vi "PCO_RecorderSaveImage_B8.vi"(0 "pImgBuf":u8[][](array[numeric])=array1x4097[4097 elements], 1 "wWidth":u16, 2 "wHeight":u16, 3 "szFilePath":path, 5 "error in (no error)":errorcluster {"code" format="%x"}, 6 "isColor":bool, 8 "bIsBitmap":bool, 9 "PCO_METADATA_STRUCT":T1, 10 "bOverwrite":bool) -> (14 "ErrorMessage":i32 format="%x", 19 "error out":errorcluster {"code" format="%x"})   [LabVIEW 2019, in "Recorder.lvlib"]
doc: "int WINAPI PCO_RecorderSaveImage(void* pImgBuf, WORD wWidth, WORD wHeight, const char* cFileType, bool bIsBitmap, const char* szFilePath, bool bOverwrite, PCO_METADATA_STRUCT* strMetadata);"
uses:
  Recorder.lvlib
  pco.sdk/Structures/Structures.lvlib
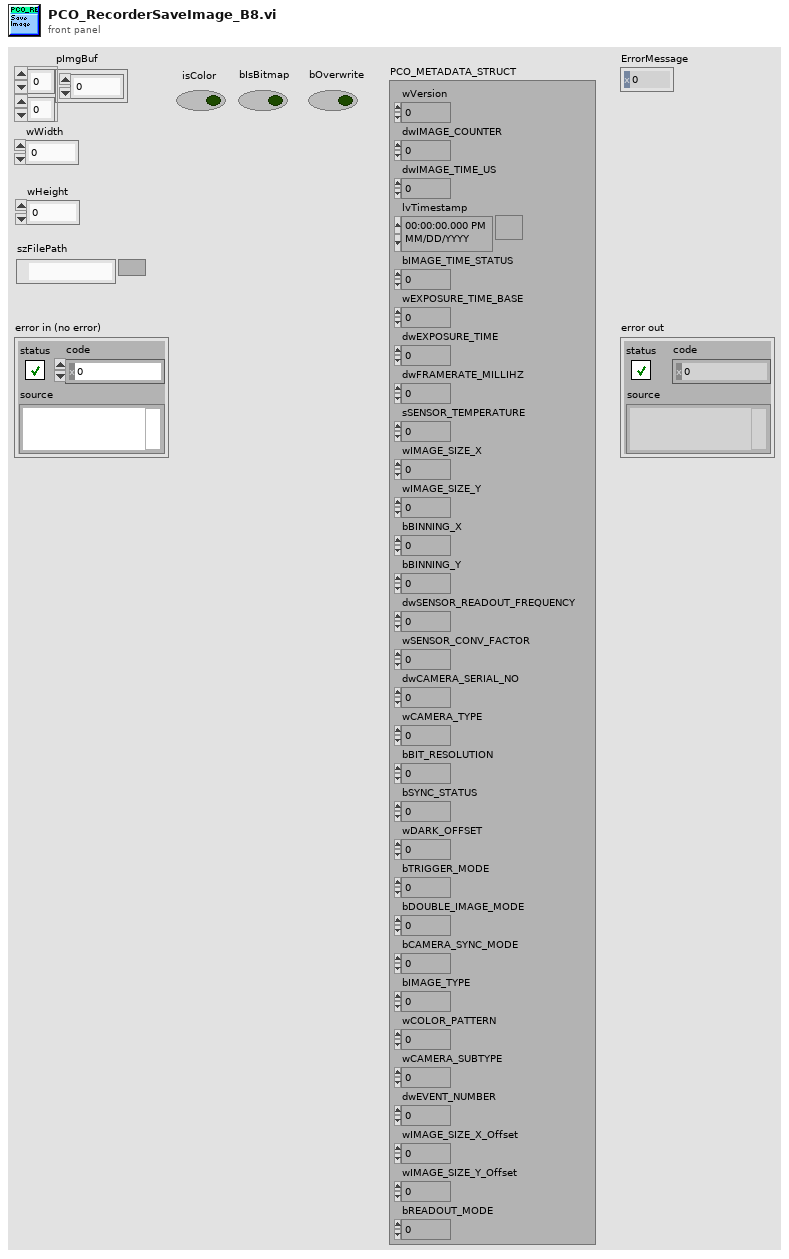
[diagram p1: front panel]
types:
  T1 = cluster{"wVersion":u16, "dwIMAGE_COUNTER":u32, "dwIMAGE_TIME_US":u32, "lvTimestamp":timestamp, "bIMAGE_TIME_STATUS":u8, "wEXPOSURE_TIME_BASE":u16, "dwEXPOSURE_TIME":u32, "dwFRAMERATE_MILLIHZ":u32, "sSENSOR_TEMPERATURE":i16, "wIMAGE_SIZE_X":u16, "wIMAGE_SIZE_Y":u16, "bBINNING_X":u8, "bBINNING_Y":u8, "dwSENSOR_READOUT_FREQUENCY":u32, "wSENSOR_CONV_FACTOR":u16, "dwCAMERA_SERIAL_NO":u32, "wCAMERA_TYPE":u16, "bBIT_RESOLUTION":u8, "bSYNC_STATUS":u8, "wDARK_OFFSET":u16, "bTRIGGER_MODE":u8, "bDOUBLE_IMAGE_MODE":u8, "bCAMERA_SYNC_MODE":u8, "bIMAGE_TYPE":u8, "wCOLOR_PATTERN":u16, "wCAMERA_SUBTYPE":u16, "dwEVENT_NUMBER":u32, "wIMAGE_SIZE_X_Offset":u16, "wIMAGE_SIZE_Y_Offset":u16, "bREADOUT_MODE":u8}
  T2 = typedef "LVDateTimeRec.ctl" = cluster{"fractional second":dbl, "second":i32, "minute":i32, "hour":i32, "day of month":i32, "month":i32, "year":i32, "day of week":i32, "day of year":i32, "DST":i32}
  T3 = cluster{"wSize":u16, "wVersion":u16, "bIMAGE_COUNTER_BCD":cluster{u8, u8, u8, u8}, "bIMAGE_TIME_US_BCD":cluster{u8, u8, u8}, "bIMAGE_TIME_SEC_BCD":u8, "bIMAGE_TIME_MIN_BCD":u8, "bIMAGE_TIME_HOUR_BCD":u8, "bIMAGE_TIME_DAY_BCD":u8, "bIMAGE_TIME_MON_BCD":u8, "bIMAGE_TIME_YEAR_BCD":u8, "bIMAGE_TIME_STATUS":u8, "wEXPOSURE_TIME_BASE":u16, "dwEXPOSURE_TIME":u32, "dwFRAMERATE_MILLIHZ":u32, "sSENSOR_TEMPERATURE":i16, "wIMAGE_SIZE_X":u16, "wIMAGE_SIZE_Y":u16, "bBINNING_X":u8, "bBINNING_Y":u8, "dwSENSOR_READOUT_FREQUENCY":u32, "wSENSOR_CONV_FACTOR":u16, "dwCAMERA_SERIAL_NO":u32, "wCAMERA_TYPE":u16, "bBIT_RESOLUTION":u8, "bSYNC_STATUS":u8, "wDARK_OFFSET":u16, "bTRIGGER_MODE":u8, "bDOUBLE_IMAGE_MODE":u8, "bCAMERA_SYNC_MODE":u8, "bIMAGE_TYPE":u8, "wCOLOR_PATTERN":u16, "wCAMERA_SUBTYPE":u16, "dwEVENT_NUMBER":u32, "wIMAGE_SIZE_X_Offset":u16, "wIMAGE_SIZE_Y_Offset":u16, "bREADOUT_MODE":u8}
  T4 = enum16{"big-endian, network order", "native, host order", "little-endian"}
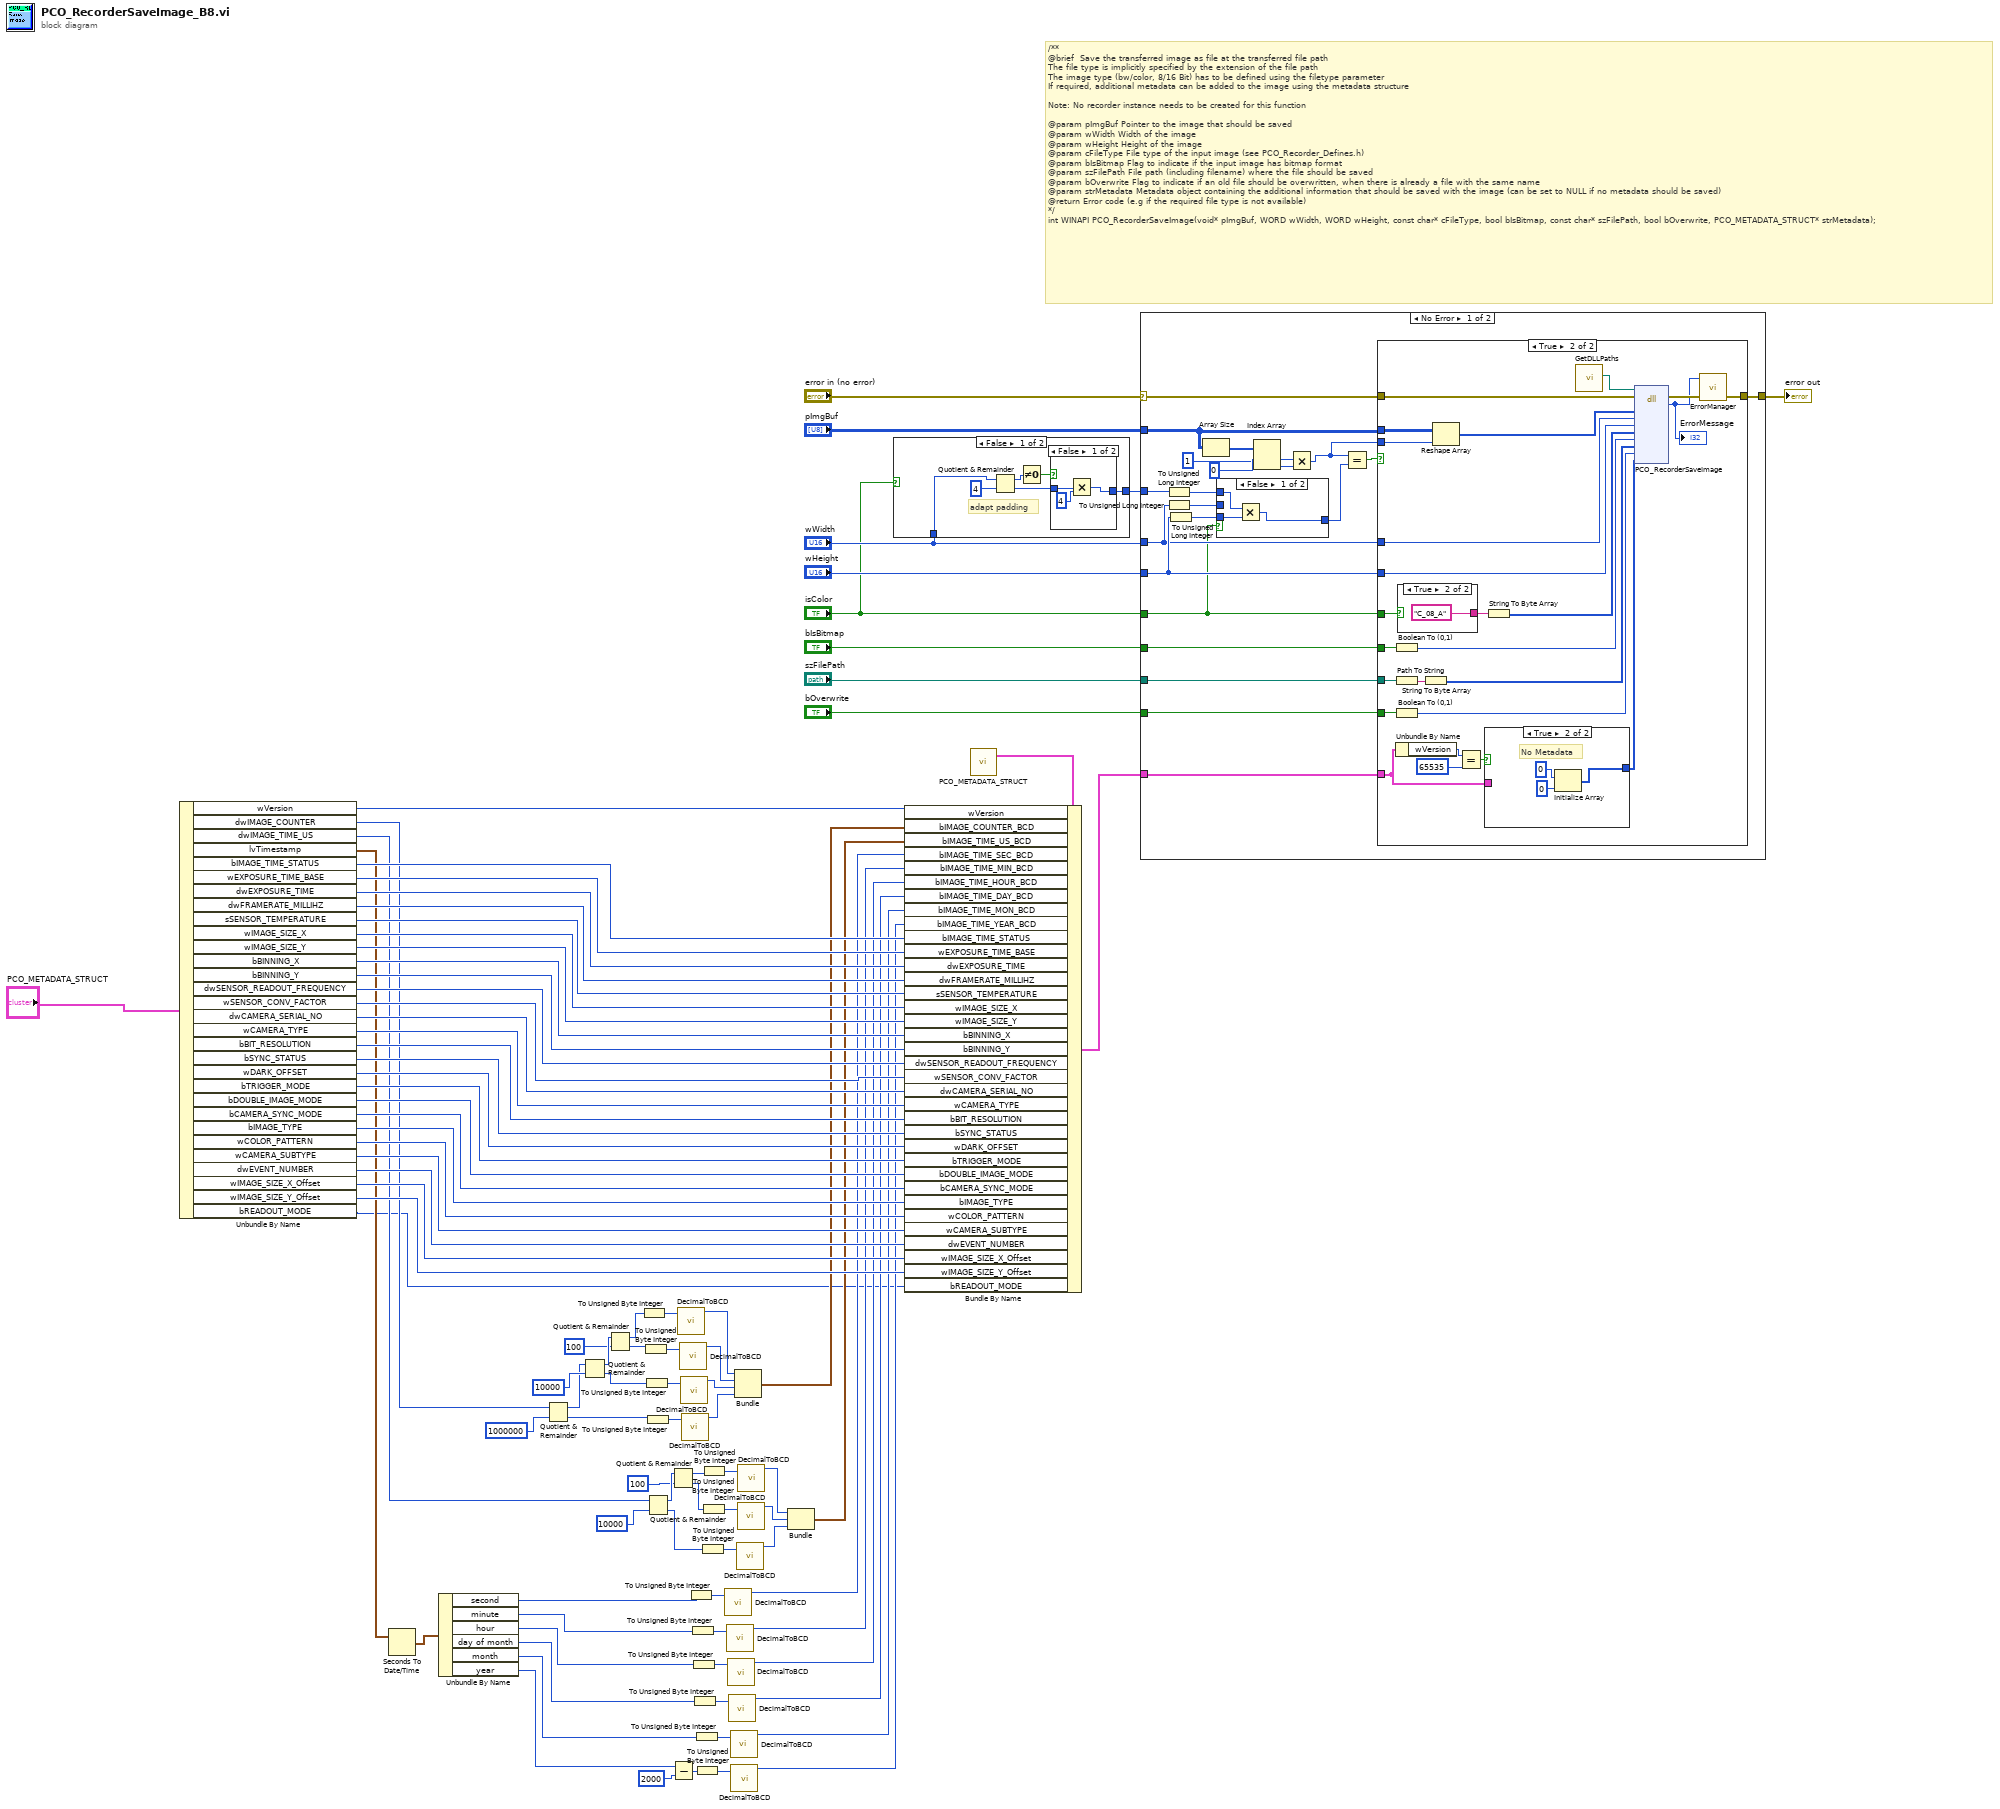
[diagram p0: block diagram]
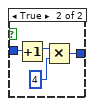
[diagram p2: hidden frame]
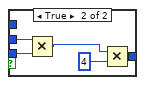
[diagram p4: hidden frame]
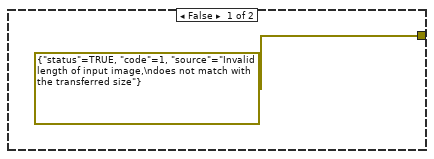
[diagram p5: hidden frame]
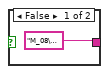
[diagram p6: hidden frame]
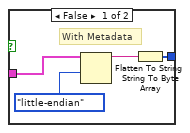
[diagram p7: hidden frame]
diagram:
  # "/**\n@brief  Save the transferred image as file at the transferred file path\nThe file type is implicitly specified by the extension of the file path\nThe image type (bw/color, 8/16 Bit) has to be defined using the filetype parameter\nIf required, additional metadata can be added to the image using the metadata structure\n\nNote: No recorder instance needs to be created for this function\n\n@param pImgBuf Pointer to the image that should be saved\n@param wWidth Width of the image\n@param wHeight Height of the image\n@param cFileType File type of the input image (see PCO_Recorder_Defines.h)\n@param bIsBitmap Flag to indicate if the input image has bitmap format\n@param szFilePath File path (including filename) where the file should be saved\n@param bOverwrite Flag to indicate if an old file should be overwritten, when there is already a file with the same name\n@param strMetadata Metadata object containing the additional information that should be saved with the image (can be set to NULL if no metadata should be saved)\n@return Error code (e.g if the required file type is not available)\n*/\nint WINAPI PCO_RecorderSaveImage(void* pImgBuf, WORD wWidth, WORD wHeight, const char* cFileType, bool bIsBitmap, const char* szFilePath, bool bOverwrite, PCO_METADATA_STRUCT* strMetadata);"
  n1 = Unbundle By Name("PCO_METADATA_STRUCT") -> ("wVersion"=w84:u16, "dwIMAGE_COUNTER"=w18:u32, "dwIMAGE_TIME_US"=w23:u32, "lvTimestamp"=w58:timestamp, "bIMAGE_TIME_STATUS"=w72:u8, "wEXPOSURE_TIME_BASE"=w59:u16, "dwEXPOSURE_TIME"=w60:u32, "dwFRAMERATE_MILLIHZ"=w61:u32, "sSENSOR_TEMPERATURE"=w62:i16, "wIMAGE_SIZE_X"=w63:u16, "wIMAGE_SIZE_Y"=w64:u16, "bBINNING_X"=w65:u8, "bBINNING_Y"=w66:u8, "dwSENSOR_READOUT_FREQUENCY"=w67:u32, "wSENSOR_CONV_FACTOR"=w68:u16, "dwCAMERA_SERIAL_NO"=w69:u32, "wCAMERA_TYPE"=w70:u16, "bBIT_RESOLUTION"=w71:u8, "bSYNC_STATUS"=w73:u8, "wDARK_OFFSET"=w74:u16, "bTRIGGER_MODE"=w75:u8, "bDOUBLE_IMAGE_MODE"=w76:u8, "bCAMERA_SYNC_MODE"=w77:u8, "bIMAGE_TYPE"=w78:u8, "wCOLOR_PATTERN"=w79:u16, "wCAMERA_SUBTYPE"=w80:u16, "dwEVENT_NUMBER"=w81:u32, "wIMAGE_SIZE_X_Offset"=w82:u16, "wIMAGE_SIZE_Y_Offset"=w83:u16, "bREADOUT_MODE"=w1:u8)
  n2 = Seconds To Date/Time(time stamp (now)=w58) -> (date time rec=w57:T2)  [unwired: 1 in]
  n3 = Unbundle By Name(w57) -> ("second"=w56:i32, "minute"=w53:i32, "hour"=w48:i32, "day of month"=w47:i32, "month"=w46:i32, "year"=w43:i32)
  n4 = Quotient & Remainder(x=w18, y=u32 1000000 ("x")) -> (x-y*floor(x/y)=w17:u32, floor(x/y)=w12:u32)
  n5 = Quotient & Remainder(x=w17, y=u32 10000 ("x")) -> (x-y*floor(x/y)=w21:u32, floor(x/y)=w11:u32)
  n6 = Quotient & Remainder(x=w21, y=u32 100 ("x")) -> (x-y*floor(x/y)=w9:u32, floor(x/y)=w10:u32)
  n7 = To Unsigned Byte Integer(number=w9) -> (unsigned 8bit integer=w16:u8)
  n8 = To Unsigned Byte Integer(number=w10) -> (unsigned 8bit integer=w15:u8)
  n9 = To Unsigned Byte Integer(number=w11) -> (unsigned 8bit integer=w14:u8)
  n10 = To Unsigned Byte Integer(number=w12) -> (unsigned 8bit integer=w13:u8)
  n11 = Quotient & Remainder(x=w23, y=u32 10000 ("x")) -> (x-y*floor(x/y)=w35:u32, floor(x/y)=w28:u32)
  n12 = Quotient & Remainder(x=w35, y=u32 100 ("x")) -> (x-y*floor(x/y)=w32:u32, floor(x/y)=w30:u32)
  n13 = Subtract(x=w43, y=2000) -> (x-y=w44:i32)
  n14 = call "DecimalToBCD.vi"("U8"=w16) -> ("BCD"=w8:u8)  [unwired: 10 in]
  n15 = call "DecimalToBCD.vi"("U8"=w15) -> ("BCD"=w7:u8)  [unwired: 10 in]
  n16 = call "DecimalToBCD.vi"("U8"=w14) -> ("BCD"=w6:u8)  [unwired: 10 in]
  n17 = call "DecimalToBCD.vi"("U8"=w13) -> ("BCD"=w5:u8)  [unwired: 10 in]
  n18 = To Unsigned Byte Integer(number=w56) -> (unsigned 8bit integer=w55:u8)
  n19 = To Unsigned Byte Integer(number=w53) -> (unsigned 8bit integer=w54:u8)
  n20 = To Unsigned Byte Integer(number=w48) -> (unsigned 8bit integer=w52:u8)
  n21 = To Unsigned Byte Integer(number=w47) -> (unsigned 8bit integer=w49:u8)
  n22 = To Unsigned Byte Integer(number=w46) -> (unsigned 8bit integer=w50:u8)
  n23 = To Unsigned Byte Integer(number=w44) -> (unsigned 8bit integer=w51:u8)
  n24 = To Unsigned Byte Integer(number=w28) -> (unsigned 8bit integer=w29:u8)
  n25 = To Unsigned Byte Integer(number=w30) -> (unsigned 8bit integer=w31:u8)
  n26 = To Unsigned Byte Integer(number=w32) -> (unsigned 8bit integer=w33:u8)
  n27 = call "DecimalToBCD.vi"("U8"=w55) -> ("BCD"=w37:u8)  [unwired: 10 in]
  n28 = call "DecimalToBCD.vi"("U8"=w54) -> ("BCD"=w38:u8)  [unwired: 10 in]
  n29 = call "DecimalToBCD.vi"("U8"=w52) -> ("BCD"=w39:u8)  [unwired: 10 in]
  n30 = call "DecimalToBCD.vi"("U8"=w49) -> ("BCD"=w40:u8)  [unwired: 10 in]
  n31 = call "DecimalToBCD.vi"("U8"=w50) -> ("BCD"=w41:u8)  [unwired: 10 in]
  n32 = call "DecimalToBCD.vi"("U8"=w51) -> ("BCD"=w42:u8)  [unwired: 10 in]
  n33 = Bundle("BCD"=w8, "BCD"=w7, "BCD"=w6, "BCD"=w5) -> (w4:cluster{"BCD":u8, "BCD":u8, "BCD":u8, "BCD":u8})  [unwired: 1 in]
  n34 = call "DecimalToBCD.vi"("U8"=w29) -> ("BCD"=w25:u8)  [unwired: 10 in]
  n35 = call "DecimalToBCD.vi"("U8"=w31) -> ("BCD"=w26:u8)  [unwired: 10 in]
  n36 = call "DecimalToBCD.vi"("U8"=w33) -> ("BCD"=w27:u8)  [unwired: 10 in]
  n37 = Bundle("BCD"=w27, "BCD"=w26, "BCD"=w25) -> (w24:cluster{"BCD":u8, "BCD":u8, "BCD":u8})  [unwired: 1 in]
  n38 = case shown="False" "isColor" {
    tunnel: "wWidth" -> [w97 w109]
    tunnel: [w96 w109] -> w87
    frame False {
      # "adapt padding"
      n39 = Quotient & Remainder(x=w97, y=u16 4) -> (x-y*floor(x/y)=w100:u16, floor(x/y)=w98:u16)
      n40 = Not Equal To 0?(x=w100) -> (x != 0?=w99:bool)
      n41 = case shown="False" w99 {
        tunnel: w98 -> [w104 w108]
        tunnel: [w102 w105] -> w96
        frame False {
          n42 = Multiply(x=w104, y=u16 4) -> (x*y=w102:u16)
        }
        frame True {
          n43 = Increment(x=w108) -> (x+1=w106:u16)
          n44 = Multiply(x=w106, y=u16 4) -> (x*y=w105:u16)
        }
      }
    }
    frame True {
    }
  }
  n45 = call "PCO_METADATA_STRUCT.vi"() -> ("PCO_METADATA_STRUCT_Raw"=w86:T3)  [unwired: 4 in, 3 out]
  n46 = Bundle By Name(cluster=w86, "wVersion"=w84, "bIMAGE_COUNTER_BCD"=w4, "bIMAGE_TIME_US_BCD"=w24, "bIMAGE_TIME_SEC_BCD"=w37, "bIMAGE_TIME_MIN_BCD"=w38, "bIMAGE_TIME_HOUR_BCD"=w39, "bIMAGE_TIME_DAY_BCD"=w40, "bIMAGE_TIME_MON_BCD"=w41, "bIMAGE_TIME_YEAR_BCD"=w42, "bIMAGE_TIME_STATUS"=w72, "wEXPOSURE_TIME_BASE"=w59, "dwEXPOSURE_TIME"=w60, "dwFRAMERATE_MILLIHZ"=w61, "sSENSOR_TEMPERATURE"=w62, "wIMAGE_SIZE_X"=w63, "wIMAGE_SIZE_Y"=w64, "bBINNING_X"=w65, "bBINNING_Y"=w66, "dwSENSOR_READOUT_FREQUENCY"=w67, "wSENSOR_CONV_FACTOR"=w68, "dwCAMERA_SERIAL_NO"=w69, "wCAMERA_TYPE"=w70, "bBIT_RESOLUTION"=w71, "bSYNC_STATUS"=w73, "wDARK_OFFSET"=w74, "bTRIGGER_MODE"=w75, "bDOUBLE_IMAGE_MODE"=w76, "bCAMERA_SYNC_MODE"=w77, "bIMAGE_TYPE"=w78, "wCOLOR_PATTERN"=w79, "wCAMERA_SUBTYPE"=w80, "dwEVENT_NUMBER"=w81, "wIMAGE_SIZE_X_Offset"=w82, "wIMAGE_SIZE_Y_Offset"=w83, "bREADOUT_MODE"=w1) -> (w85:T3)
  n47 = case shown="No Error" "error in (no error)" {
    selector: "error in (no error)" -> [w130 w175]
    tunnel: "pImgBuf" -> [w129 _]
    tunnel: "wWidth" -> [w116 _]
    tunnel: "wHeight" -> [w117 _]
    tunnel: "bIsBitmap" -> [w123 _]
    tunnel: [w131 w175] -> w92
    tunnel: "szFilePath" -> [w124 _]
    tunnel: "bOverwrite" -> [w125 _]
    tunnel: "isColor" -> [w111 _]
    tunnel: w85 -> [w126 _]
    tunnel: w87 -> [w115 _]
    frame No Error {
      n48 = To Unsigned Long Integer(number=w115) -> (unsigned 32bit integer=w114:u32)
      n49 = To Unsigned Long Integer(number=w116) -> (unsigned 32bit integer=w113:u32)
      n50 = To Unsigned Long Integer(number=w117) -> (unsigned 32bit integer=w112:u32)
      n51 = Array Size(array=w129) -> (size(s)=w122:i32[])
      n52 = case shown="False" w111 {
        tunnel: [w132 w138] -> w128
        tunnel: w114 -> [w133 _]
        tunnel: w113 -> [_ w136]
        tunnel: w112 -> [w134 w137]
        frame False {
          n53 = Multiply(x=w133, y=w134) -> (x*y=w132:u32)
        }
        frame True {
          n54 = Multiply(x=w136, y=w137) -> (x*y=w135:u32)
          n55 = Multiply(x=w135, y=u32 4) -> (x*y=w138:u32)
        }
      }
      n56 = Index Array(array=w122, index #1=u32 0 ("index"), index #2=u32 1 ("index")) -> (element #1=w118:i32, element #2=w119:i32)
      n57 = Multiply(x=w118, y=w119) -> (x*y=w110:u32)
      n58 = Equal?(x=w110, y=w128) -> (x = y?=w127:bool)
      n59 = case shown="True" w127 {
        tunnel: w129 -> [_ w143]
        tunnel: w116 -> [_ w165]
        tunnel: w117 -> [_ w164]
        tunnel: w123 -> [_ w163]
        tunnel: [errorcluster {"status"=TRUE, "code"=1, "source"="Invalid length of input image,\ndoes not match with the transferred size"} ("error out") w157] -> w131
        tunnel: w130 -> [_ w160]
        tunnel: w111 -> [_ w149]
        tunnel: w126 -> [_ w151]
        tunnel: w125 -> [_ w150]
        tunnel: w124 -> [_ w147]
        tunnel: w110 -> [_ w141]
        frame False {
        }
        frame True {
          n60 = Boolean To (0,1)(Boolean=w163) -> (0, 1=w162:i16)
          n61 = Path To String(path=w147) -> (string=w148:string)
          n62 = Boolean To (0,1)(Boolean=w150) -> (0, 1=w161:i16)
          n63 = Unbundle By Name(w151) -> ("wVersion"=w155:u16)
          n64 = case shown="True" w149 {
            tunnel: ["M_08\u0000" "C_08_A"] -> w145
            frame False {
            }
            frame True {
            }
          }
          n65 = String To Byte Array(string=w148) -> (unsigned byte array=w146:u8[])
          n66 = Reshape Array(w143, w141) -> (w142:u8[])
          n67 = Equal?(x=w155, y=u16 65535) -> (x = y?=w153:bool)
          n68 = case shown="True" w153 {
            tunnel: [w169 w172] -> w152
            tunnel: w151 -> [w170 _]
            frame False {
              # "With Metadata"
              n69 = Flatten To String(anything=w170, byte order (0:big-endian, network order)=T4."little-endian" ("Byte-Reihenfolge (0:Big-Endian, Netzwerkreihenfolge)")) -> (data string=w171:string)  [unwired: 2 in, 2 out]
              n70 = String To Byte Array(string=w171) -> (unsigned byte array=w169:u8[])
            }
            frame True {
              # "No Metadata"
              n71 = Initialize Array(u8 0, 0 ("dimension size")) -> (w172:u8[])
            }
          }
          n72 = String To Byte Array(string=w145) -> (unsigned byte array=w144:u8[])
          n73 = call "GetDLLPaths.vi"() -> ("PCO_Recorder_Path"=w159:path)  [unwired: 8 in, 3 out]
          n74 = dll-call lib="?" fn="PCO_RecorderSaveImage"(path in=w159, error in=w160, "pImgBuf"=w142, "wWidth"=w165, "wHeight"=w164, "cFileType"=w144, "bIsBitmap"=w162, "szFilePath"=w146, "bOverwrite"=w161, "strMetadata"=w152) -> (error out=w158:errorcluster, "return type"=w156:i32)  [unwired: 9 in, 1 out]
          "ErrorMessage" <- w156
          n75 = call "ErrorManager.vi"("error in (no error)"=w158, "error code"=w156) -> ("error out"=w157:errorcluster)  [unwired: 2 in, 1 out]
        }
      }
    }
    frame Error {
    }
  }
  "error out" <- w92
